vi "NodeToUse.vi"(0 "reference in":refnum<class "AbstractNode.lvclass">, 3 "reference in 2":refnum<class "AbstractNode.lvclass">, 5 "error in (no error)":errorcluster) -> (14 "reference out":refnum<class "AbstractNode.lvclass">, 15 "Same":bool, 17 "reference out 2":refnum<class "AbstractNode.lvclass">, 19 "error out":errorcluster)   [LabVIEW 2016, in "AbstractNode.lvclass"]
uses:
  <resource>/Framework/Providers/Open_GDS/UML/AbstractNode_class/AbstractNode.lvclass
  <resource>/Framework/Providers/Open_GDS/UML/AbstractNode_class/AbstractNode.lvclass/AbstractNode.ctl
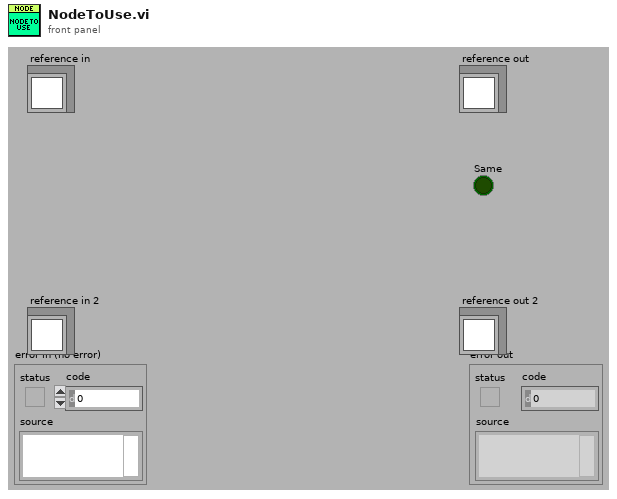
[diagram p1: front panel]
types:
  T1 = typedef "AbstractNode.lvclass/ObjectAttributes.ctl" = cluster{"parent":refnum<class "AbstractNode.lvclass">, "children":refnum<class "AbstractNode.lvclass">[], "Hidden":bool}
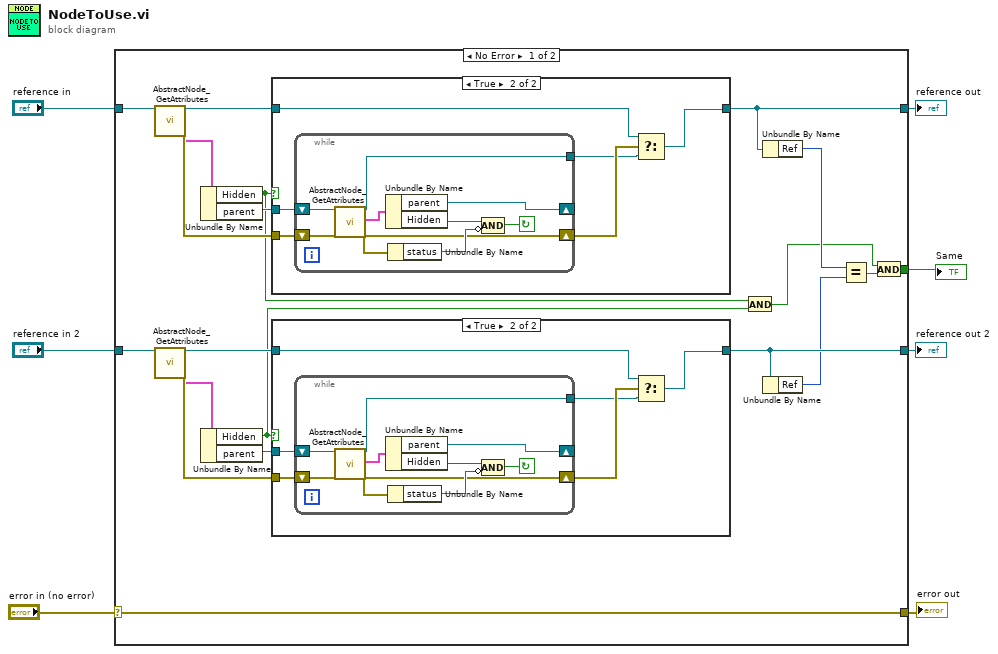
[diagram p0: block diagram]
diagram:
  n1 = case shown="No Error" "error in (no error)" {
    selector: "error in (no error)" -> [w19 w62]
    tunnel: [w19 w62] -> w6
    tunnel: [w18 w61] -> w4
    tunnel: "reference in" -> [w27 w61]
    tunnel: [w17 w60] -> w3
    tunnel: "reference in 2" -> [w20 w60]
    tunnel: [w10 _] -> w1
    frame No Error {
      n2 = call <resource>:"AbstractNode_GetAttributes.vi"("reference in"=w27) -> ("reference out"=w24:refnum<class "AbstractNode.lvclass">, "Data"=w8:T1, "error out"=w25:errorcluster)  [unwired: 15 in, 1 out]
      n3 = call <resource>:"AbstractNode_GetAttributes.vi"("reference in"=w20) -> ("reference out"=w23:refnum<class "AbstractNode.lvclass">, "Data"=w9:T1, "error out"=w22:errorcluster)  [unwired: 15 in, 1 out]
      n4 = Unbundle By Name(w8) -> ("Hidden"=w13:bool, "parent"=w26:refnum<class "AbstractNode.lvclass">)
      n5 = Unbundle By Name(w9) -> ("Hidden"=w12:bool, "parent"=w21:refnum<class "AbstractNode.lvclass">)
      n6 = case shown="True" w13 {
        tunnel: w26 -> [_ w50]
        tunnel: w25 -> [_ w49]
        tunnel: w24 -> [w44 w45]
        tunnel: [w44 w47] -> w18
        frame False {
        }
        frame True {
          n7 = while {
            shift-right: [w57] -> _
            shift-left: w50 -> [w59]
            shift-right: [w54] -> w48
            shift-left: w49 -> [w58]
            tunnel: [w52] -> w46
            stop <- w53 continue-if-true
            n8 = call <resource>:"AbstractNode_GetAttributes.vi"("reference in"=w59, "error in (no error)"=w58) -> ("reference out"=w52:refnum<class "AbstractNode.lvclass">, "Data"=w51:T1, "error out"=w54:errorcluster)  [unwired: 14 in, 1 out]
            n9 = Unbundle By Name(w51) -> ("parent"=w57:refnum<class "AbstractNode.lvclass">, "Hidden"=w56:bool)
            n10 = Unbundle By Name(w54) -> ("status"=w55:bool)
            n11 = Compound Arithmetic op=AND(w56, invert w55) -> (w53:bool)
          }
          n12 = Select(t=w45, s=w48, f=w46) -> (s? t:f=w47:refnum<class "AbstractNode.lvclass">)
        }
      }
      n13 = case shown="True" w12 {
        tunnel: w21 -> [_ w34]
        tunnel: w22 -> [_ w33]
        tunnel: w23 -> [w28 w29]
        tunnel: [w28 w31] -> w17
        frame False {
        }
        frame True {
          n14 = while {
            shift-right: [w41] -> _
            shift-left: w34 -> [w43]
            shift-right: [w38] -> w32
            shift-left: w33 -> [w42]
            tunnel: [w36] -> w30
            stop <- w37 continue-if-true
            n15 = call <resource>:"AbstractNode_GetAttributes.vi"("reference in"=w43, "error in (no error)"=w42) -> ("reference out"=w36:refnum<class "AbstractNode.lvclass">, "Data"=w35:T1, "error out"=w38:errorcluster)  [unwired: 14 in, 1 out]
            n16 = Unbundle By Name(w35) -> ("parent"=w41:refnum<class "AbstractNode.lvclass">, "Hidden"=w40:bool)
            n17 = Unbundle By Name(w38) -> ("status"=w39:bool)
            n18 = Compound Arithmetic op=AND(w40, invert w39) -> (w37:bool)
          }
          n19 = Select(t=w29, s=w32, f=w30) -> (s? t:f=w31:refnum<class "AbstractNode.lvclass">)
        }
      }
      n20 = And(x=w13, y=w12) -> (x .and. y?=w11:bool)
      n21 = Unbundle By Name(w18) -> ("Ref"=w15:u32)
      n22 = Unbundle By Name(w17) -> ("Ref"=w16:u32)
      n23 = Equal?(x=w15, y=w16) -> (x = y?=w14:bool)
      n24 = And(x=w11, y=w14) -> (x .and. y?=w10:bool)
    }
    frame Error {
    }
  }
  "error out" <- w6
  "reference out" <- w4
  "reference out 2" <- w3
  "Same" <- w1
